vi "selectionSort.vi"() -> ()   [LabVIEW 2014]
panel:
  out "Waveform Graph":dbl[](graph)
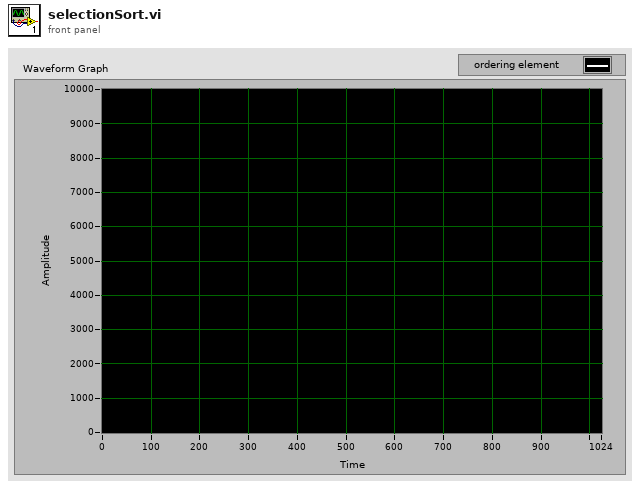
[diagram p1: front panel]
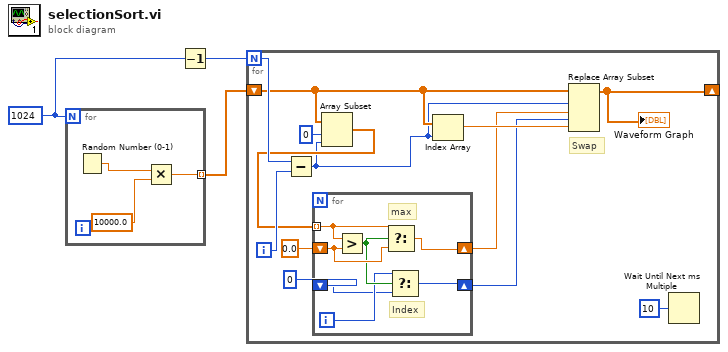
[diagram p0: block diagram]
diagram:
  w1 = 1024
  n1 = for {
    N: w1 -> [_]
    tunnel: [w4] -> w3 mode=indexing
    n2 = Random Number (0-1)() -> (number: 0 to 1=w6:dbl)
    n3 = Multiply(x=w6, y=10000.0) -> (x*y=w4:dbl)
  }
  n4 = Decrement(x=w1) -> (x-1=w2:i32)
  n5 = for {
    N: w2 -> [w18]
    shift-right: [w7] -> _
    shift-left: w3 -> [w16]
    i -> [w17]
    # "Swap"
    n6 = Subtract(x=w18, y=w17) -> (x-y=w8:i32)
    n7 = Array Subset(array=w16, index=0, length=w8) -> (w13:dbl[])
    n8 = for {
      tunnel: w13 -> [w26] mode=indexing
      shift-right: [w24] -> w10
      shift-left: 0.0 -> [w25]
      shift-right: [w23] -> w9
      shift-left: 0 -> [w20]
      i -> [w21]
      # "Index"
      # "max"
      n9 = Greater?(x=w26, y=w25) -> (0:w22:bool)
      n10 = Select(t=w26, s=w22, f=w25) -> (s? t:f=w24:dbl)
      n11 = Select(t=w21, s=w22, f=w20) -> (s? t:f=w23:i32)
    }
    n12 = Index Array(array=w16, index=w8) -> (element=w15:dbl)
    n13 = Replace Array Subset(array=w16, new element #1=w10, index #1=w8, new element #2=w15, index #2=w9) -> (w7:dbl[])
    "Waveform Graph" <- w7
    n14 = Wait Until Next ms Multiple(millisecond multiple=u32 10) -> ()  [unwired: 1 out]
  }
